vi "spietro_exponential.vi"() -> ()   [LabVIEW 2010]
uses:
  <vilib>/Utility/file.llb/Write To Spreadsheet File (DBL).vi
  <vilib>/Analysis/NI_AALBase.lvlib
panel:
  in  "Save?":bool
  out "XY Graph":T1(graph)
  in  "Histogram Intervals":i32
  out "Exponential Distribution":dbl[](graph)
  in  "Expected Random Numbers":dbl
  in  "Number of Iterations":i32
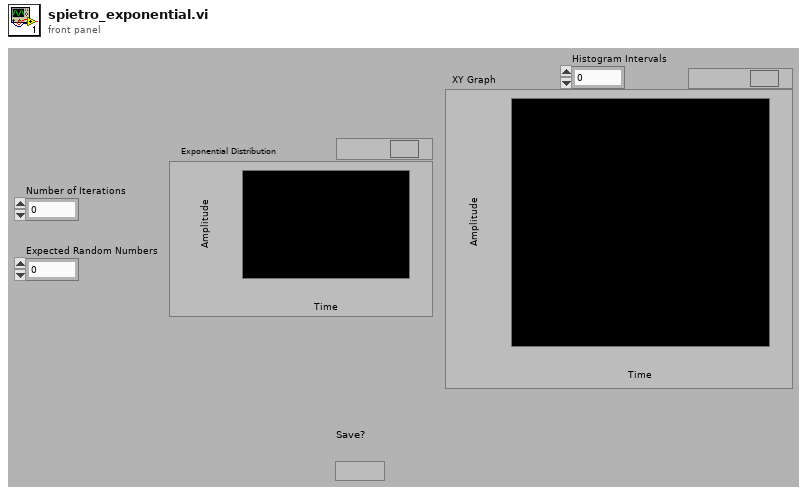
[diagram p1: front panel]
types:
  T1 = cluster{"X Values":dbl[], "Histogram: h(x)":i32[]}
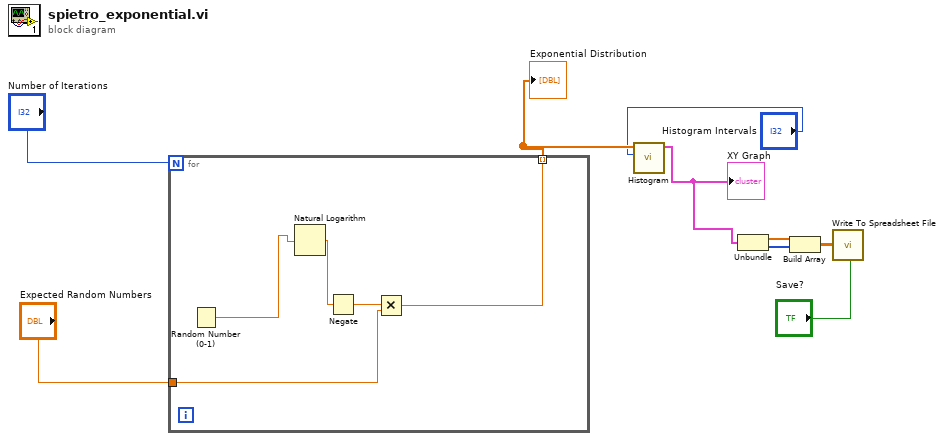
[diagram p0: block diagram]
diagram:
  n1 = for {
    N: "Number of Iterations" -> [_]
    tunnel: "Expected Random Numbers" -> [w14]
    tunnel: [w12] -> w7 mode=indexing
    n2 = Random Number (0-1)() -> (number: 0 to 1=w11:dbl)
    n3 = Natural Logarithm(1:w11) -> (0:w10:dbl)
    n4 = Negate(x=w10) -> (-x=w13:dbl)
    n5 = Multiply(x=w13, y=w14) -> (x*y=w12:dbl)
  }
  "Exponential Distribution" <- w7
  n6 = call <vilib>:"Histogram.vi"("intervals"="Histogram Intervals", "X"=w7) -> ("Histogram Graph"=w5:T1)  [unwired: 6 in, 3 out]
  "XY Graph" <- w5
  n7 = Unbundle(w5) -> ("X Values"=w4:dbl[], "Histogram: h(x)"=w3:i32[])
  n8 = Build Array(w4, w3) -> (w2:dbl[][])
  n9 = call-poly <vilib>:"Write To Spreadsheet File.vi"("transpose? (no:F)"="Save?", "2D data"=w2) -> ()  [unwired: 6 in, 1 out]
